vi "Unpack For Grpc.vi"(8 "error in (no error)":errorcluster, 9 "Configuration / Resuls (Config)":enum16{"Configuration", "Results"}(ring), 10 "Any":T1, 11 "MeasurementPluginService in":refnum<class "MeasurementPluginService.lvclass">) -> (0 "error out":errorcluster, 2 "Data Value":variant, 3 "MeasurementPluginService in":refnum<class "MeasurementPluginService.lvclass">)   [LabVIEW 2020, in "MeasurementLink Measurement Server.lvlib" / "MeasurementPluginService.lvclass"]
uses:
  MeasurementPluginService.lvclass
  <vilib>/gRPC/LabVIEW gRPC Library/Shared/Any.ctl
  MeasurementLink gRPC Utilities/Error Strings Global.vi
  MeasurementLink gRPC Utilities/MeasurementLink gRPC Utilities.lvlib
  <vilib>/gRPC/LabVIEW gRPC Library/grpc-lvsupport-release.lvlib
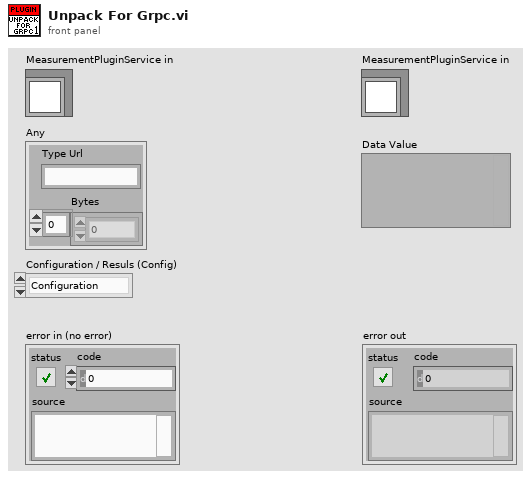
[diagram p1: front panel]
types:
  T1 = typedef "grpc-lvsupport-release.lvlib/Any.ctl" = cluster{"Type Url":string, "Bytes":u8[]}
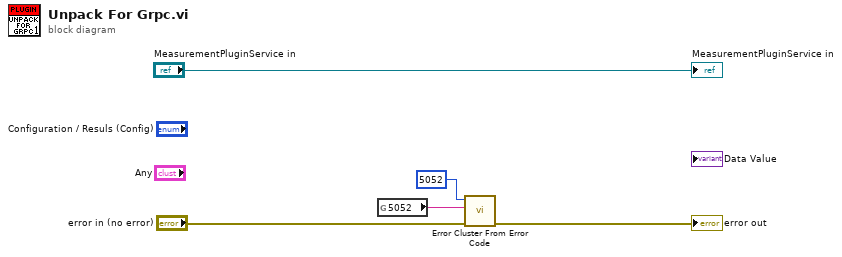
[diagram p0: block diagram]
diagram:
  n1 = global read "Error Strings Global.vi" "5052"() -> (w1:string)
  n2 = call <vilib>:"Error Cluster From Error Code.vi"("error in (no error)"="error in (no error)", "error message (\"\")"=w1, "error code (0)"=5052) -> ("error out"=→"error out":errorcluster)  [unwired: 6 in]
  "MeasurementPluginService in" <- "MeasurementPluginService in"
